vi "Prelog_SubVI.vi"() -> (2 "new file path (Not A Path if cancelled)":path)   [LabVIEW 2012]
uses:
  <vilib>/Utility/file.llb/Write To Spreadsheet File (string).vi
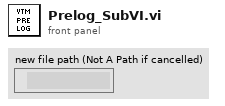
[diagram p1: front panel]
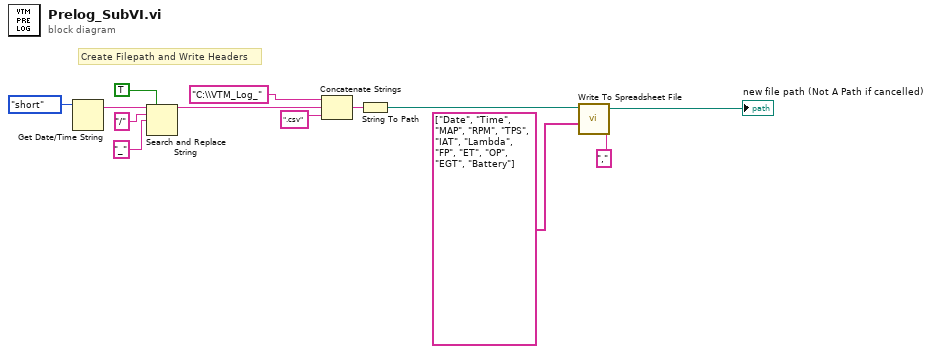
[diagram p0: block diagram]
diagram:
  # "Create Filepath and Write Headers"
  n1 = Get Date/Time String(date format (0)=enum16{"short", "long", "abbreviated"}."short") -> (date string=w2:string)  [unwired: 2 in, 1 out]
  n2 = Search and Replace String(replace all?=TRUE ("replace all? (F)"), input string=w2, search string="/", replace string="_" ("replace string (\"\")")) -> (result string=w6:string)  [unwired: 4 in, 3 out]
  n3 = Concatenate Strings("C:\\VTM_Log_", w6, ".csv" ("string")) -> (w8:string)
  n4 = String To Path(string=w8) -> (path=w10:path)
  n5 = call-poly <vilib>:"Write To Spreadsheet File.vi"("delimiter (\\t)"="," ("delimiter (\\t)"), "1D data"=string[] ["Date", "Time", "MAP", "RPM", "TPS", "IAT", "Lambda", "FP", "ET", "OP", "EGT", "Battery"], "file path (dialog if empty)"=w10) -> ("new file path (Not A Path if cancelled)"=→"new file path (Not A Path if cancelled)":path)  [unwired: 5 in]
